vi "Read License String.vi"(8 "error in (no error)":errorcluster) -> (0 "error out":errorcluster, 3 "License String":string)   [LabVIEW 2015, in "Add License to VI Documentation.lvlib"]
uses:
  Add License to VI Documentation.lvlib
  <vilib>/Utility/error.llb/Error Cluster From Error Code.vi
  <vilib>/ErrorRing/Error Ring.xnode
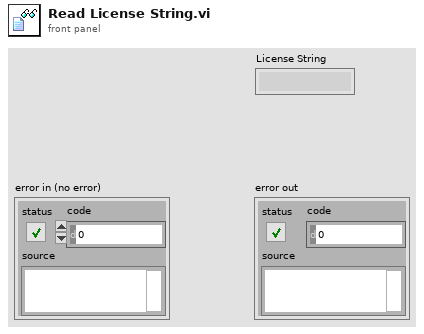
[diagram p1: front panel]
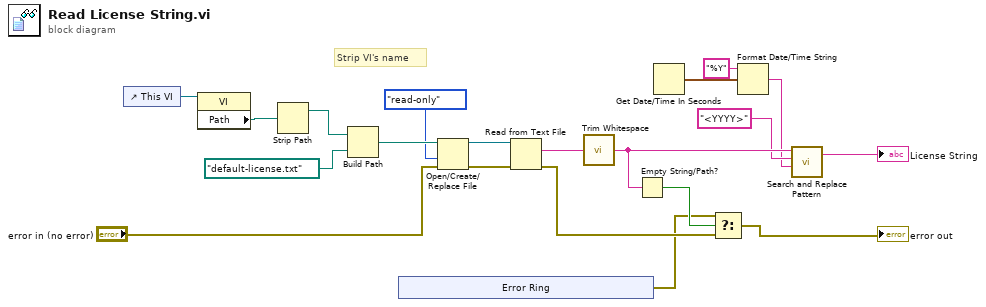
[diagram p0: block diagram]
diagram:
  # "Strip VI's name"
  n1 = control-ref of="This VI"() -> (w13:refnum<vi>)
  n2 = property class="VI"(reference=w13) -> ("Path"=w12:path)  [unwired: 1 in, 2 out]
  n3 = Strip Path(path=w12) -> (stripped path=w11:path)  [unwired: 1 out]
  n4 = Build Path(base path=w11, name or relative path=path "default-license.txt") -> (appended path=w19:path)
  n5 = xnode "Error Ring"() -> ("error out"=w8:errorcluster)
  n6 = Open/Create/Replace File(file path (use dialog)=w19, error in="error in (no error)", access (0:read/write)=enum16{"read/write", "read-only", "write-only"}."read-only") -> (refnum out=w17:refnum<file>, error out=w16:errorcluster)  [unwired: 3 in, 1 out]
  n7 = Read from Text File(file (use dialog)=w17, error in=w16) -> (text=w14:string, error out=w9:errorcluster)  [unwired: 2 in, 2 out]
  n8 = call <vilib>:"Trim Whitespace.vi"("string"=w14) -> ("trimmed string"=w6:string)  [unwired: 1 in]
  n9 = Empty String/Path?(string/path=w6) -> (empty?=w10:bool)
  n10 = Get Date/Time In Seconds() -> (seconds since 1Jan1904=w3:timestamp)
  n11 = Select(t=w8, s=w10, f=w9) -> (s? t:f=→"error out":errorcluster)
  n12 = Format Date/Time String(time format string (%c)="%Y", seconds (now)=w3) -> (date/time string=w1:string)  [unwired: 1 in]
  n13 = call <vilib>:"Search and Replace Pattern.vi"("string"=w6, "regular expression (\"\")"="<YYYY>" ("regular expression (\"\")"), "replace string (\"\")"=w1) -> ("result string"=→"License String":string)  [unwired: 2 in, 1 out]
